vi "New Dialog.vi"(8 "error in (no error)":errorcluster, 11 "Item Ref in":T17 format="%.0x") -> (0 "error out":errorcluster, 3 "Item Ref out":T17 format="%.0x")   [LabVIEW 2019, in "DSF System Explorer.lvlib"]
uses:
  DSF System Explorer.lvlib
  DSF Core.lvlibp/Typedefs/DSF Version Info.ctl
  <vilib>/NI VeriStand/Custom Device API/Custom Device Item Ref.ctl
  <vilib>/NI VeriStand/Custom Device API/Custom Device API.lvlib
  DSF Core.lvlibp/Typedefs/DSF Timing Info.ctl
  DSF Core.lvlibp/Typedefs/Core Plugin Configuration.ctl
  DSF Core.lvlibp/Typedefs/DSF Settings Info.ctl
  DSF Core.lvlibp/Typedefs/Core Thread Configuration.ctl
  DSF Core.lvlibp/Typedefs/DSF Direction.ctl
  DSF Core.lvlibp/Typedefs/DSF Timeout Behavior.ctl
  DSF Core.lvlibp/Typedefs/Core Group Configuration.ctl
  DSF Core.lvlibp/Typedefs/Core Transfer Configuration.ctl
  DSF Core.lvlibp/Typedefs/DSF Data Type.ctl
  DSF Core.lvlibp/Typedefs/Core Channel Configuration.ctl
  DSF Core.lvlibp/Typedefs/DSF Engine Channel Configuration.ctl
  DSF Core.lvlibp/Typedefs/DSF Engine Transfer Configuration.ctl
  DSF Core.lvlibp/Typedefs/DSF Engine Transfer Group Configuration.ctl
  DSF Core.lvlibp/Typedefs/DSF Engine Plugin Thread Configuration.ctl
  DSF Core.lvlibp/Typedefs/DSF Engine Plugin Configuration.ctl
  DSF Core.lvlibp/Typedefs/DSF Engine Framework Configuration.ctl
panel:
  in  "framework configuration":T1={"plugins"=[{"core"={"name"="Plugin", "components"=[], "cycle timing"={"priority"=10000, "decimation"=1, "offset"=0}}, "component settings"=[], "threads"=[{"core"={"processor"=-2, "priority offset"=0}, "component settings"=[], "transfer groups"=[{"core"={"name"="Group", "direction"=enum."Tx", "cycle timing"={"priority"=100, "decimation"=1, "offset"=0}, "timeout behavior"=enum."Increment Late Count", "enable conversion"=FALSE}, "component settings"=[], "transfers"=[{"core"={"name"="Transfer"}, "component settings"=[], "channels"=[{"core"={"name"="Channel", "units"="V", "engine data type"=enum."DBL", "string data type"=enum."DBL", "string offset"=0}, "component settings"=[]}]}]}]}]}]}
  out "Duration":u32 format="%d ms"
  in  "Apply":bool
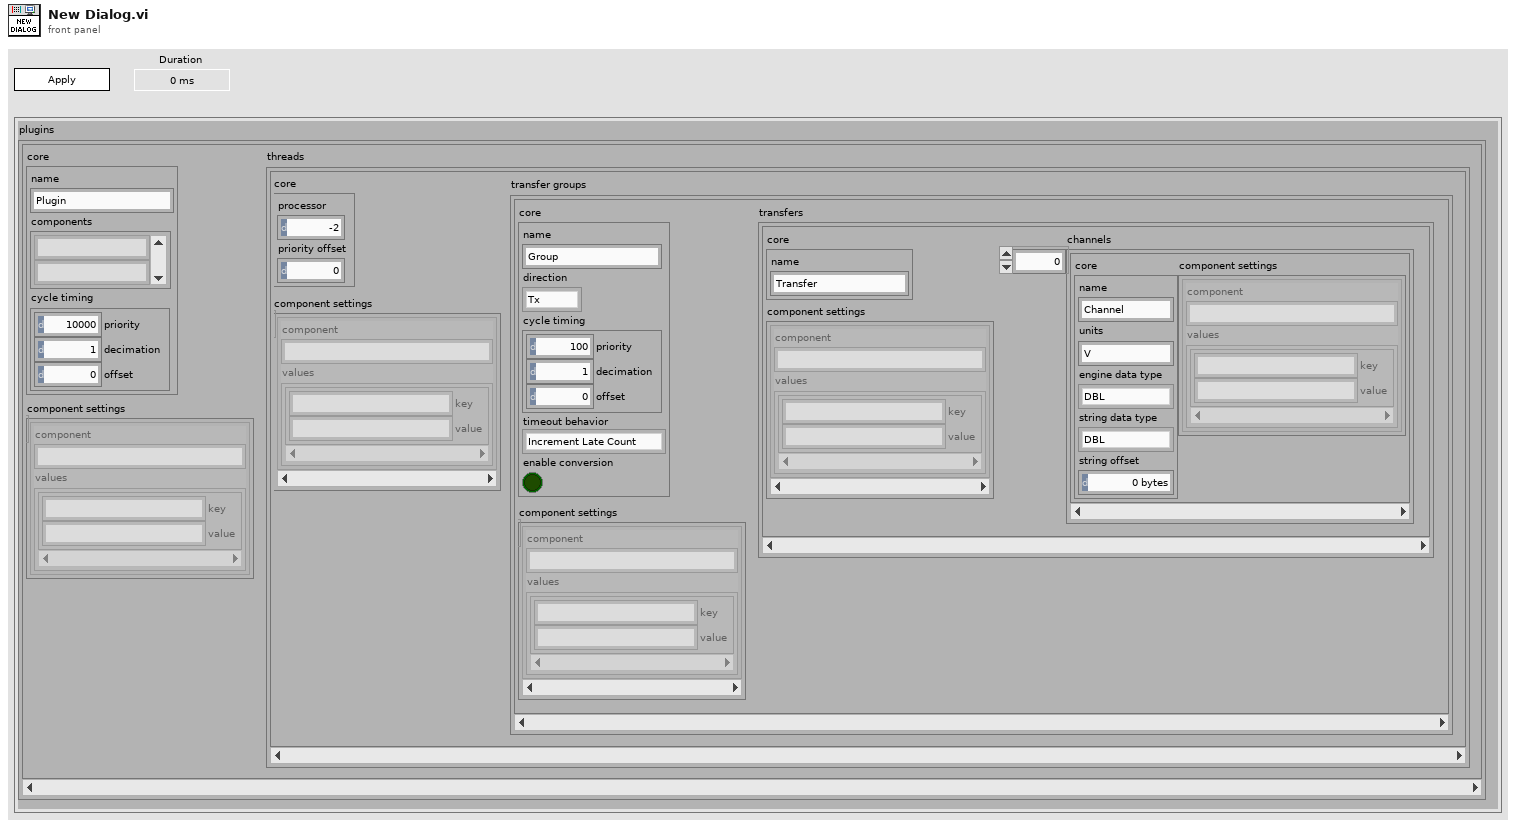
[diagram p1: front panel]
types:
  T1 = typedef "DSF Core.lvlibp/DSF Engine Framework Configuration.ctl" = cluster{"plugins":T2[]}
  T2 = typedef "DSF Core.lvlibp/DSF Engine Plugin Configuration.ctl" = cluster{"core":T3, "component settings":T5[], "threads":T6[]}
  T3 = typedef "DSF Core.lvlibp/Plugin Configuration.lvclass/Core Plugin Configuration.ctl" = cluster{"name":string, "components":string[], "cycle timing":T4}
  T4 = typedef "DSF Core.lvlibp/DSF Timing Info.ctl" = cluster{"priority":u64, "decimation":u64, "offset":u64}
  T5 = typedef "DSF Core.lvlibp/DSF Settings Info.ctl" = cluster{"component":string, "values":cluster{"key":string, "value":string}[]}
  T6 = typedef "DSF Core.lvlibp/DSF Engine Plugin Thread Configuration.ctl" = cluster{"core":T7, "component settings":T5[], "transfer groups":T8[]}
  T7 = typedef "DSF Core.lvlibp/Thread Configuration.lvclass/Core Thread Configuration.ctl" = cluster{"processor":i32, "priority offset":i16}
  T8 = typedef "DSF Core.lvlibp/DSF Engine Transfer Group Configuration.ctl" = cluster{"core":T9, "component settings":T5[], "transfers":T12[]}
  T9 = typedef "DSF Core.lvlibp/Group Configuration.lvclass/Core Group Configuration.ctl" = cluster{"name":string, "direction":T10, "cycle timing":T4, "timeout behavior":T11, "enable conversion":bool}
  T10 = typedef "DSF Core.lvlibp/DSF Direction.ctl" = enum8{"Tx", "Rx"}
  T11 = typedef "DSF Core.lvlibp/DSF Timeout Behavior.ctl" = enum8{"Increment Late Count", "Throw Error"}
  T12 = typedef "DSF Core.lvlibp/DSF Engine Transfer Configuration.ctl" = cluster{"core":T13, "component settings":T5[], "channels":T14[]}
  T13 = typedef "DSF Core.lvlibp/Transfer Configuration.lvclass/Core Transfer Configuration.ctl" = cluster{"name":string}
  T14 = typedef "DSF Core.lvlibp/DSF Engine Channel Configuration.ctl" = cluster{"core":T15, "component settings":T5[]}
  T15 = typedef "DSF Core.lvlibp/Channel Configuration.lvclass/Core Channel Configuration.ctl" = cluster{"name":string, "units":string, "engine data type":T16, "string data type":T16, "string offset":u64}
  T16 = typedef "DSF Core.lvlibp/DSF Data Type.ctl" = enum8{"Bool", "SGL", "DBL", "I8", "I16", "I32", "I64", "U8", "U16", "U32", "U64"}
  T17 = typedef "Custom Device API.lvlib/Custom Device Item Ref.ctl" = u64
  T18 = typedef "DSF Core.lvlibp/DSF Version Info.ctl" = cluster{"major":u32, "minor":u32, "fix":u32, "build":string}
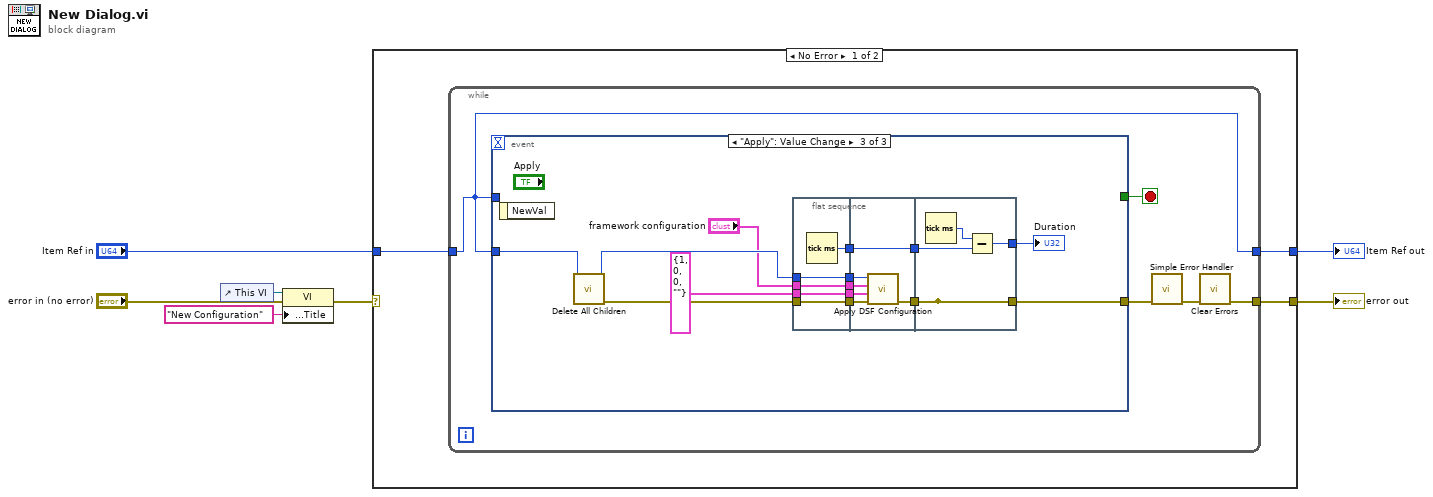
[diagram p0: block diagram]
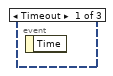
[diagram p2: hidden frame]
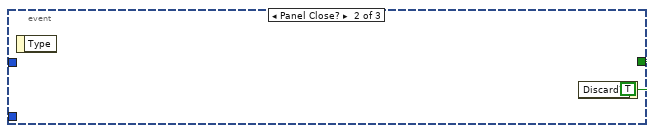
[diagram p3: hidden frame]
diagram:
  n1 = control-ref of="This VI"() -> (w4:refnum<vi>)
  n2 = property class="VI"(reference=w4, error in="error in (no error)", "Front Panel.Title"="New Configuration" ("Front Panel Window:Title")) -> (error out=w1:errorcluster)  [unwired: 1 out]
  n3 = case shown="No Error" w1 {
    selector: w1 -> [_ w46]
    tunnel: [w10 w46] -> w7
    tunnel: "Item Ref in" -> [w9 w47]
    tunnel: [w8 w47] -> w5
    frame No Error {
      n4 = while {
        tunnel: w9 -> [w11]
        tunnel: [w11] -> w8
        tunnel: [w14] -> w10
        stop <- w15 stop-if-true
        n5 = event shown="[2] \"Apply\": Value Change" {
          selector: _ -> [_ _ _]
          dyn-events: _ -> [_ _ _]
          timeout: _ -> [_ _ _]
          tunnel: [_ w16 _] -> w15
          tunnel: [_ _ w24] -> w13
          tunnel: w11 -> [_ _ w21]
          tunnel: w11 -> [_ _ _]
          event Timeout {
            n6 = event-data() -> ()  [unwired: 1 in, 1 out]
          }
          event Panel Close? {
            w16 = TRUE ("Discard?")
            n7 = event-data() -> ()  [unwired: 1 in, 1 out]
            n8 = event-data("Discard?"=w16) -> ()  [unwired: 1 in, 1 out]
          }
          event "Apply": Value Change {
            n9 = event-data() -> ()  [unwired: 1 in, 1 out]
            n10 = call "Delete All Children.vi"("Item Ref in"=w21) -> ("error out"=w19:errorcluster, "Item Ref out"=w20:T17)  [unwired: 9 in]
            n11 = flat-sequence {
              tunnel: [w35] -> w30
              tunnel: "framework configuration" -> [w34]
              tunnel: [w34] -> w26
              tunnel: w20 -> [w33]
              tunnel: [w33] -> w25
              tunnel: w19 -> [w32]
              tunnel: [w32] -> w23
              tunnel: T18 {"major"=1, "minor"=0, "fix"=0, "build"=""} ("version") -> [w31]
              tunnel: [w31] -> w22
              tunnel: w30 -> [w41]
              tunnel: [w41] -> w29
              tunnel: [w38] -> w27
              tunnel: w26 -> [w40]
              tunnel: w25 -> [w39]
              tunnel: w23 -> [w37]
              tunnel: w22 -> [w36]
              tunnel: w29 -> [w45]
              tunnel: [w43] -> w28
              tunnel: w27 -> [w42]
              tunnel: [w42] -> _
              tunnel: [w42] -> w24
              frame #0 {
                n12 = Tick Count (ms)() -> (millisecond timer value=w35:u32)
              }
              frame #1 {
                n13 = call "Apply DSF Configuration.vi"("error in (no error)"=w37, "version"=w36, "framework configuration"=w40, "Item Ref in"=w39) -> ("error out"=w38:errorcluster)  [unwired: 7 in]
              }
              frame #2 {
                n14 = Tick Count (ms)() -> (millisecond timer value=w44:u32)
                n15 = Subtract(x=w44, y=w45) -> (x-y=w43:u32)
              }
            }
            "Duration" <- w28
          }
        }
        n16 = call <vilib>:"Simple Error Handler.vi"("error in (no error)"=w13) -> ("error out"=w12:errorcluster)  [unwired: 4 in, 4 out]
        n17 = call <vilib>:"Clear Errors.vi"("error in (no error)"=w12) -> ("error out"=w14:errorcluster)  [unwired: 5 in, 1 out]
      }
    }
    frame Error {
    }
  }
  "Item Ref out" <- w5
  "error out" <- w7
